vi "Flatten to JSON.vi"(8 "error in (no error)":errorcluster, 11 "Test Scope in":refnum<class "Test Scope.lvclass">) -> (0 "error out":errorcluster, 1 "JSON Data":string, 2 "Version":string, 3 "Test Scope out":refnum<class "Test Scope.lvclass">)   [LabVIEW 2015, in "Test Scope.lvclass"]
uses:
  Test Scope.lvclass
  Test Scope.lvclass/Test Scope.ctl
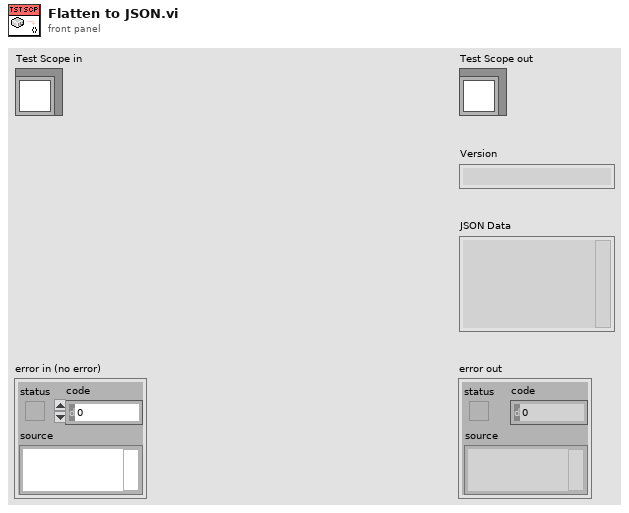
[diagram p1: front panel]
types:
  T1 = typedef "Test Scope.lvclass/JSON Data.ctl" = cluster{"V/div":dbl, "V Offset":dbl, "s/div":dbl, "s offset":dbl, "trigger level":dbl}
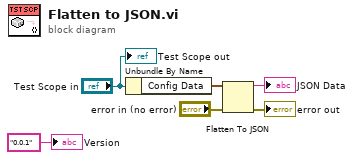
[diagram p0: block diagram]
diagram:
  n1 = Unbundle By Name("Test Scope in") -> ("Config Data"=w4:T1)
  n2 = Flatten To JSON(anything=w4, error in (no error)="error in (no error)") -> (JSON string=→"JSON Data":string, 11:→"error out":errorcluster)  [unwired: 1 in]
  "Test Scope out" <- "Test Scope in"
  "Version" <- "0.0.1" ("Version")
